vi "Get_reference_samplingdata.vi"(0 "SPU":refnum<k24>, 1 "STSProcess.ILSTS":refnum<k24>, 2 "Refdata_struct":refnum<k24>[](array[refnum]), 5 "Ref_monitordata_struct":refnum<k24>[](array[refnum]), 7 "MPM":refnum<k24>[](array[refnum]), 9 "TSL":refnum<k24>, 11 "错误输入（无错误）":errorcluster) -> (6 "ILSTS out":refnum<k24>, 15 "error out":errorcluster)   [LabVIEW 2017]
doc: "Get logging reference data & add in"
uses:
  D:/test/ILSTS/LV_IL/LV_IL_Sample_x64/DLL/STSProcess.dll
  DLL/STSProcess.dll
  D:/test/ILSTS/LV_IL/LV_IL_Sample_x64/DLL/InstrumentDLL.dll
  DLL/InstrumentDLL.dll
  Share/PowerMonitorType.vi
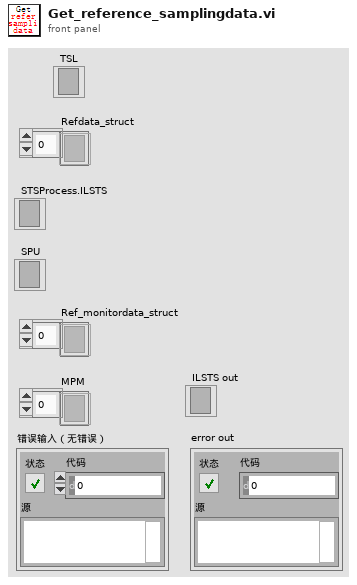
[diagram p1: front panel]
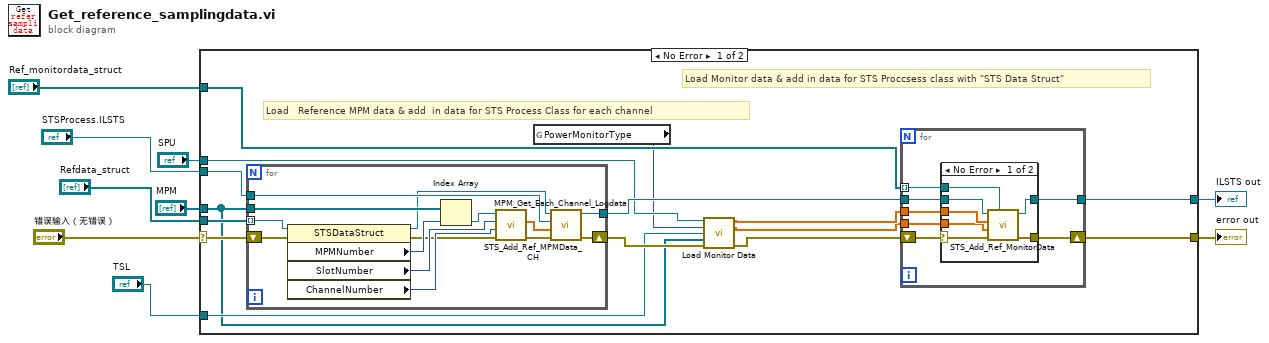
[diagram p0: block diagram]
diagram:
  n1 = case shown="No Error" "错误输入（无错误）" {
    selector: "错误输入（无错误）" -> [w21 w56]
    tunnel: "STSProcess.ILSTS" -> [w20 w55]
    tunnel: "Ref_monitordata_struct" -> [w24 _]
    tunnel: "SPU" -> [w14 _]
    tunnel: "MPM" -> [w10 _]
    tunnel: "Refdata_struct" -> [w23 _]
    tunnel: [w22 w56] -> w4
    tunnel: [w18 w55] -> w2
    tunnel: "TSL" -> [w11 _]
    frame No Error {
      # "Load Monitor data & add in data for STS Proccsess class with \"STS Data Struct\""
      # "Load　Reference MPM data & add  in data for STS Process Class for each channel"
      n2 = for {
        tunnel: w23 -> [w49] mode=indexing
        tunnel: w10 -> [w52]
        tunnel: w20 -> [w50]
        shift-right: [w48] -> w13
        shift-left: w21 -> [w46]
        tunnel: [w41] -> w19
        n3 = property on="属性节点" class="STSDataStruct"(reference=w49, error in=w46) -> (reference out=w42:refnum<k24>, error out=w47:errorcluster, "MPMNumber"=w51:i32, "SlotNumber"=w54:i32, "ChannelNumber"=w53:i32)
        n4 = Index Array(array=w52, index=w51) -> (element=w45:refnum<k24>)
        n5 = call "MPM_Get_Each_Channel_Logdata.vi"("error in (no error)"=w47, "channelNumber"=w53, "moduleNumber"=w54, ".NET Reference in"=w45) -> ("error out"=w43:errorcluster, "data out"=w44:sgl[])  [unwired: 5 in, 1 out]
        n6 = call "STS_Add_Ref_MPMData_CH.vi"("错误输入（无错误）"=w43, "data"=w44, "STSProcess.ILSTS"=w50, "Setting"=w42) -> ("错误输出"=w48:errorcluster, "ILSTS"=w41:refnum<k24>)  [unwired: 6 in]
      }
      n7 = global read "PowerMonitorType.vi" "PowerMonitorType"() -> (w12:enum16{"DAQ", "MPM_220", "TSL_LOGG"})
      n8 = call "Load Monitor Data.vi"("SPU"=w14, "PowerMonitorType"=w12, "TSL"=w11, "MPM"=w10, "error in (no error)"=w13) -> ("trigger"=w17:sgl[], "monitor"=w16:sgl[], "error out"=w15:errorcluster)  [unwired: 8 in]
      n9 = for {
        tunnel: w24 -> [w30] mode=indexing
        tunnel: w19 -> [w31]
        tunnel: w17 -> [w29]
        tunnel: w16 -> [w28]
        shift-right: [w26] -> w22
        shift-left: w15 -> [w27]
        tunnel: [w25] -> w18
        n10 = case shown="No Error" w27 {
          selector: w27 -> [w34 w40]
          tunnel: w31 -> [w38 w39]
          tunnel: w30 -> [w37 _]
          tunnel: w29 -> [w36 _]
          tunnel: w28 -> [w35 _]
          tunnel: [w33 w40] -> w26
          tunnel: [w32 w39] -> w25
          frame No Error {
            n11 = call "STS_Add_Ref_MonitorData.vi"("setting"=w37, "错误输入（无错误）"=w34, "monitorData"=w35, "triggerIndex"=w36, "STSProcess.ILSTS"=w38) -> ("错误输出"=w33:errorcluster, "ILSTS out"=w32:refnum<k24>)  [unwired: 5 in]
          }
          frame Error {
          }
        }
      }
    }
    frame Error {
    }
  }
  "error out" <- w4
  "ILSTS out" <- w2
